vi "Update Active Room Details.vi"(0 "Rooms Manager Model in":refnum<class "Rooms Manager Model.lvclass">, 11 "error in (no error)":errorcluster) -> (4 "Rooms Manager Model out":refnum<class "Rooms Manager Model.lvclass">, 15 "error out":errorcluster)   [LabVIEW 2023, in "Rooms Manager Model.lvlib" / "Rooms Manager Model.lvclass"]
uses:
  Rooms Manager Model.lvclass
  Rooms Manager Model.lvclass/Rooms Manager Model.ctl
  Rooms Manager UI/Rooms Manager UI Messages/Update Active Room Details Msg/Update Active Room Details Msg.lvclass/Update Active Room Details Msg.ctl
  <vilib>/ActorFramework/Message Enqueuer/Message Enqueuer.lvclass/Message Enqueuer.ctl
  <vilib>/ActorFramework/Message Enqueuer/Enqueue.vi
  Rooms Manager UI/Rooms Manager UI Messages/Update Active Room Details Msg/Update Active Room Details Msg.lvclass
  C:/Program Files/National Instruments/LabVIEW 2023/vi.lib/ActorFramework/Message/Message.lvclass
  <vilib>/ActorFramework/Message Priority Queue/Priority Enqueue.vi
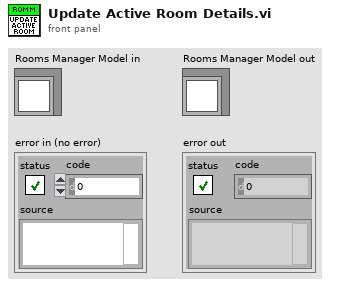
[diagram p1: front panel]
types:
  T1 = typedef "Central Data Manager.lvlib/Central Data Manager.lvclass/Room Details.ctl" = cluster{"Room No":string, "Room Size":string, "Room Occupancy Status":T2, "Guest Details":T3, "Occupancy Count (Adult)":u32, "Occupancy Count (Children)":u32, "Check-in Time":timestamp, "Check-out Time":timestamp}
  T2 = typedef "Central Data Manager.lvlib/Central Data Manager.lvclass/Room Occupancy Status.ctl" = enum16{"Not Occupied", "Occupied", "Under Maintainance", "Not Servicable"}
  T3 = typedef "Central Data Manager.lvlib/Central Data Manager.lvclass/Guest Details.ctl" = cluster{"Contact Number":string, "Primary Guest Name":string}
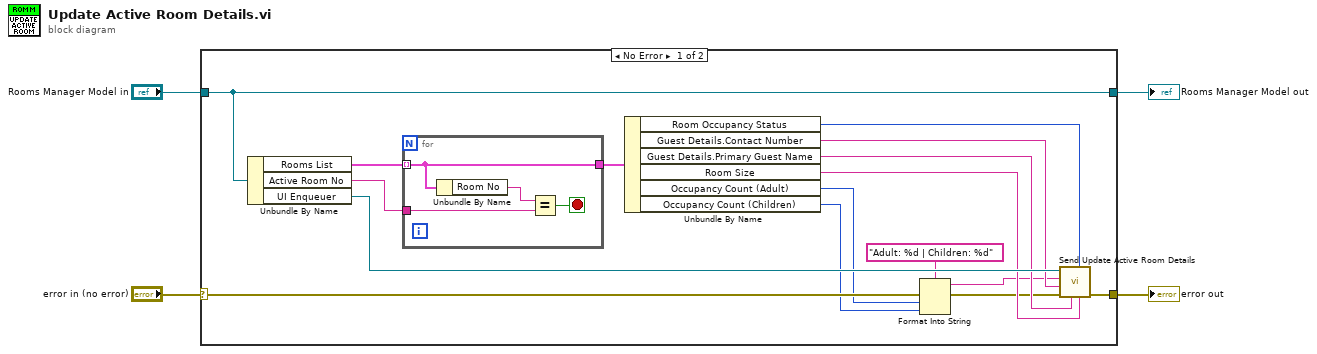
[diagram p0: block diagram]
diagram:
  n1 = case shown="No Error" "error in (no error)" {
    selector: "error in (no error)" -> [w15 w26]
    tunnel: [w14 w26] -> w3
    tunnel: [w20 w25] -> w1
    tunnel: "Rooms Manager Model in" -> [w20 w25]
    frame No Error {
      n2 = Unbundle By Name(w20) -> ("Rooms List"=w19:T1[], "Active Room No"=w18:string, "UI Enqueuer"=w16:refnum<class "Message Enqueuer.lvclass">)
      n3 = for {
        tunnel: w19 -> [w21] mode=indexing
        tunnel: w18 -> [w24]
        tunnel: [w21] -> w17
        stop <- w22 stop-if-true
        n4 = Unbundle By Name(w21) -> ("Room No"=w23:string)
        n5 = Equal?(x=w23, y=w24) -> (x = y?=w22:bool)
      }
      n6 = Unbundle By Name(w17) -> ("Room Occupancy Status"=w13:T2, "Guest Details.Contact Number"=w10:string, "Guest Details.Primary Guest Name"=w11:string, "Room Size"=w12:string, "Occupancy Count (Adult)"=w6:u32, "Occupancy Count (Children)"=w5:u32)
      n7 = Format Into String(format string="Adult: %d | Children: %d", error in=w15, w6, w5) -> (resulting string=w8:string, error out=w9:errorcluster)  [unwired: 1 in]
      n8 = call "Send Update Active Room Details.vi"("Room Size"=w12, "Status"=w13, "Guest Name"=w11, "error in (no error)"=w9, "Contact Number"=w10, "Count"=w8, "Message Enqueuer"=w16) -> ("error out"=w14:errorcluster)  [unwired: 3 in, 1 out]
    }
    frame Error {
    }
  }
  "error out" <- w3
  "Rooms Manager Model out" <- w1
